vi "DataManager.vi"(6 "DataFunction":T2, 8 "error in (no error)":errorcluster, 11 "CData In":T1) -> (0 "error out":errorcluster, 3 "CData Out":T1)   [LabVIEW 2014]
uses:
  Controls/DataFunction.ctl
  Controls/CData Core Control.ctl
  GlobalLock/Controls/GL Functions.ctl
  Class/CData.lvclass
panel:
  # "Data Manager"
  # "INPUTS"
  # "OUTPUTS"
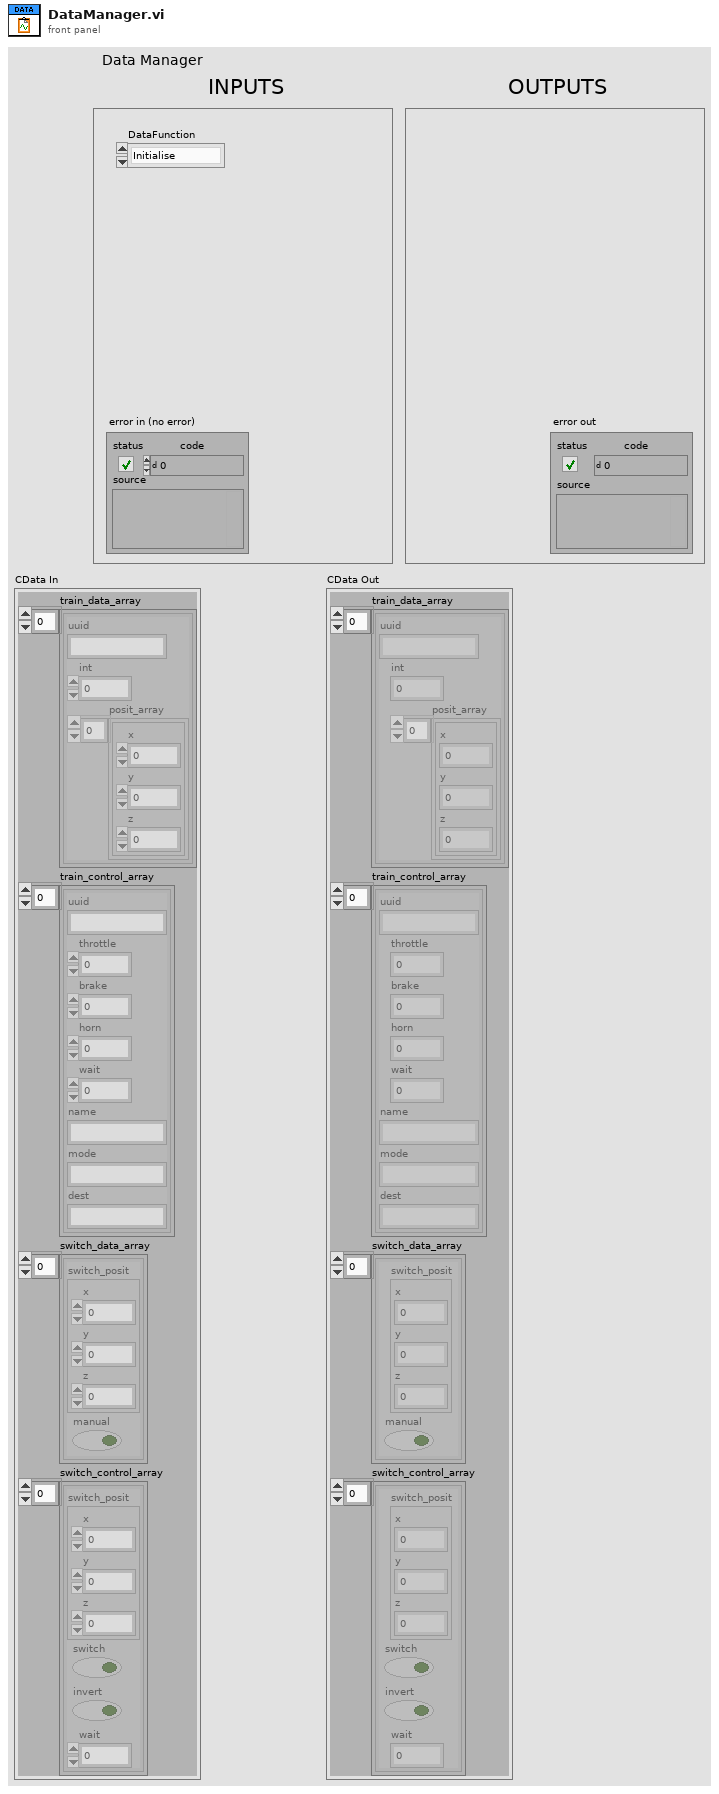
[diagram p1: front panel]
types:
  T1 = typedef "CData Core Control.ctl" = cluster{"train_data_array":cluster{"uuid":string, "int":i32, "posit_array":cluster{"x":dbl, "y":dbl, "z":dbl}[]}[], "train_control_array":cluster{"uuid":string, "throttle":dbl, "brake":dbl, "horn":dbl, "wait":dbl, "name":string, "mode":string, "dest":string}[], "switch_data_array":cluster{"switch_posit":cluster{"x":dbl, "y":dbl, "z":dbl}, "manual":bool}[], "switch_control_array":cluster{"switch_posit":cluster{"x":dbl, "y":dbl, "z":dbl}, "switch":bool, "invert":bool, "wait":dbl}[]}
  T2 = typedef "DataFunction.ctl" = enum16{"Initialise", "Release", "Get Data", "Set Data", "Preview Data"}
  T3 = typedef "GL Functions.ctl" = enum16{"Initialise", "Get", "Set", "Dispose", "Query"}
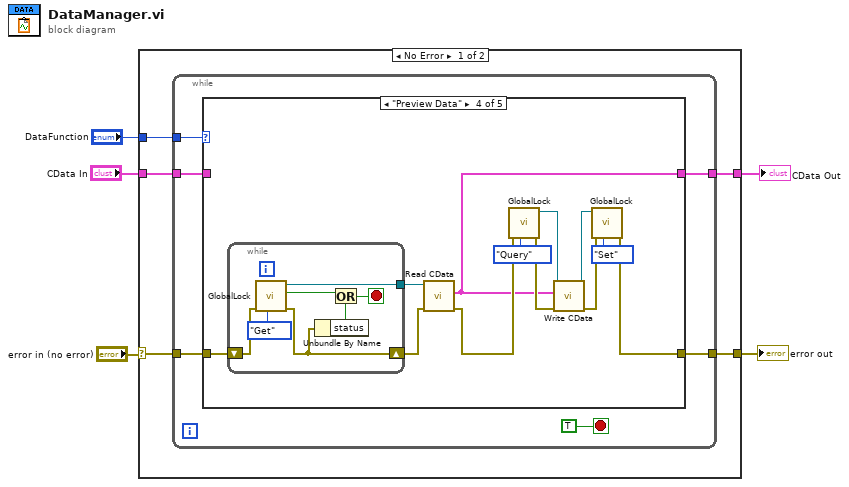
[diagram p0: block diagram]
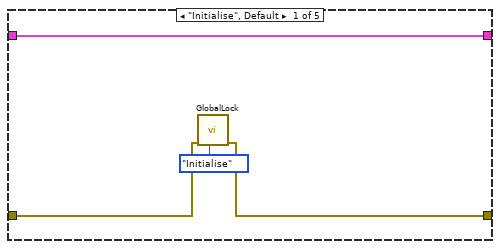
[diagram p2: hidden frame]
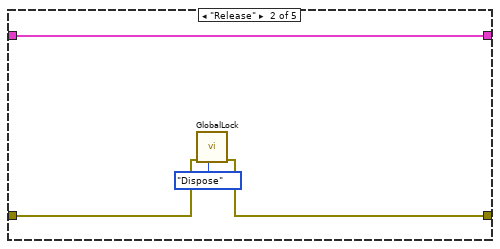
[diagram p3: hidden frame]
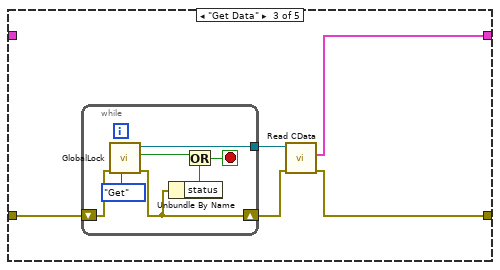
[diagram p4: hidden frame]
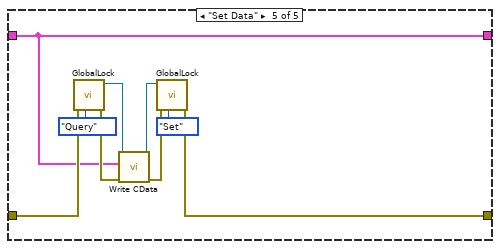
[diagram p5: hidden frame]
diagram:
  n1 = case shown="No Error" "error in (no error)" {
    selector: "error in (no error)" -> [w10 w65]
    tunnel: "DataFunction" -> [w9 _]
    tunnel: "CData In" -> [w8 w66]
    tunnel: [w7 w66] -> w2
    tunnel: [w6 w65] -> w1
    frame No Error {
      n2 = while {
        tunnel: w10 -> [w11]
        tunnel: w9 -> [w15]
        tunnel: w8 -> [w14]
        tunnel: [w13] -> w7
        tunnel: [w12] -> w6
        stop <- TRUE stop-if-true
        n3 = case shown="\"Preview Data\"" w15 {
          tunnel: w14 -> [w17 w24 _ _ w56]
          tunnel: [w17 w24 w25 w37 w56] -> w13
          tunnel: [w18 w22 w26 w38 w57] -> w12
          tunnel: w11 -> [w19 w23 w29 w48 w60]
          frame "Initialise", Default {
            n4 = call "GlobalLock.vi"("GL Functions"=GL_Functions."Initialise", "error in (no error)"=w19) -> ("error out"=w18:errorcluster)  [unwired: 7 in, 2 out]
          }
          frame "Release" {
            n5 = call "GlobalLock.vi"("GL Functions"=GL_Functions."Dispose", "error in (no error)"=w23) -> ("error out"=w22:errorcluster)  [unwired: 7 in, 2 out]
          }
          frame "Get Data" {
            n6 = while {
              shift-right: [w32] -> w27
              shift-left: w29 -> [w36]
              tunnel: [w30] -> w28
              stop <- w33 stop-if-true
              n7 = call "GlobalLock.vi"("GL Functions"=GL_Functions."Get", "error in (no error)"=w36) -> ("error out"=w32:errorcluster, "Locked?"=w34:bool, "CData Out"=w30:refnum<class "CData.lvclass">)  [unwired: 7 in]
              n8 = Unbundle By Name(w32) -> ("status"=w31:bool)
              n9 = Or(x=w34, y=w31) -> (x .or. y?=w33:bool)
            }
            n10 = call-dynamic "Read CData.vi"("error in (no error)"=w27, "CData in"=w28) -> ("error out"=w26:errorcluster, "CData"=w25:T1)  [unwired: 7 in, 1 out]
          }
          frame "Preview Data" {
            n11 = while {
              shift-right: [w51] -> w46
              shift-left: w48 -> [w55]
              tunnel: [w49] -> w47
              stop <- w52 stop-if-true
              n12 = call "GlobalLock.vi"("GL Functions"=GL_Functions."Get", "error in (no error)"=w55) -> ("error out"=w51:errorcluster, "Locked?"=w53:bool, "CData Out"=w49:refnum<class "CData.lvclass">)  [unwired: 7 in]
              n13 = Unbundle By Name(w51) -> ("status"=w50:bool)
              n14 = Or(x=w53, y=w50) -> (x .or. y?=w52:bool)
            }
            n15 = call-dynamic "Read CData.vi"("error in (no error)"=w46, "CData in"=w47) -> ("error out"=w39:errorcluster, "CData"=w37:T1)  [unwired: 7 in, 1 out]
            n16 = call "GlobalLock.vi"("GL Functions"=GL_Functions."Query", "error in (no error)"=w39) -> ("error out"=w44:errorcluster, "CData Out"=w42:refnum<class "CData.lvclass">)  [unwired: 7 in, 1 out]
            n17 = call-dynamic "Write CData.vi"("error in (no error)"=w44, "CData"=w37, "CData in"=w42) -> ("error out"=w45:errorcluster, "CData out"=w43:refnum<class "CData.lvclass">)  [unwired: 7 in]
            n18 = call "GlobalLock.vi"("GL Functions"=GL_Functions."Set", "error in (no error)"=w45, "CData In"=w43) -> ("error out"=w38:errorcluster)  [unwired: 6 in, 2 out]
          }
          frame "Set Data" {
            n19 = call "GlobalLock.vi"("GL Functions"=GL_Functions."Query", "error in (no error)"=w60) -> ("error out"=w59:errorcluster, "CData Out"=w62:refnum<class "CData.lvclass">)  [unwired: 7 in, 1 out]
            n20 = call-dynamic "Write CData.vi"("error in (no error)"=w59, "CData"=w56, "CData in"=w62) -> ("error out"=w58:errorcluster, "CData out"=w61:refnum<class "CData.lvclass">)  [unwired: 7 in]
            n21 = call "GlobalLock.vi"("GL Functions"=GL_Functions."Set", "error in (no error)"=w58, "CData In"=w61) -> ("error out"=w57:errorcluster)  [unwired: 6 in, 2 out]
          }
        }
      }
    }
    frame Error {
    }
  }
  "error out" <- w1
  "CData Out" <- w2
